vi "GE 5565PIORC.PIO.Scalar.vi"(11 "data type":T1) -> (0 "error out":errorcluster, 3 "pass?":bool)   [LabVIEW 2020]
uses:
  Typedefs/GE 5565PIORC.Data Types.ctl
  Source/GE 5565PIORC.lvclass/GE 5565PIORC.ctl
  Source/Methods/GE 5565PIORC.PIO.Write (Bool).vi
  Source/Methods/GE 5565PIORC.PIO.Read (Bool).vi
  Source/Methods/GE 5565PIORC.PIO.Write (SGL).vi
  Source/Methods/GE 5565PIORC.PIO.Read (SGL).vi
  Source/Methods/GE 5565PIORC.PIO.Write (DBL).vi
  Source/Methods/GE 5565PIORC.PIO.Read (DBL).vi
  Source/Methods/GE 5565PIORC.PIO.Write (I8).vi
  Source/Methods/GE 5565PIORC.PIO.Read (I8).vi
  Source/Methods/GE 5565PIORC.PIO.Write (I16).vi
  Source/Methods/GE 5565PIORC.PIO.Read (I16).vi
  Source/Methods/GE 5565PIORC.PIO.Write (I32).vi
  Source/Methods/GE 5565PIORC.PIO.Read (I32).vi
  Source/Methods/GE 5565PIORC.PIO.Write (I64).vi
  Source/Methods/GE 5565PIORC.PIO.Read (I64).vi
  Source/Methods/GE 5565PIORC.PIO.Write (U8).vi
  Source/Methods/GE 5565PIORC.PIO.Read (U8).vi
  Source/Methods/GE 5565PIORC.PIO.Write (U16).vi
  Source/Methods/GE 5565PIORC.PIO.Read (U16).vi
  Source/Methods/GE 5565PIORC.PIO.Write (U32).vi
  Source/Methods/GE 5565PIORC.PIO.Read (U32).vi
  Source/Methods/GE 5565PIORC.PIO.Write (U64).vi
  Source/Methods/GE 5565PIORC.PIO.Read (U64).vi
  Source/Methods/GE 5565PIORC.VISA.Move Out.vi
  Source/Methods/GE 5565PIORC.VISA.Move Out.String (U8).vi
  Source/Methods/GE 5565PIORC.VISA.Move In.vi
  Source/Methods/GE 5565PIORC.VISA.Move In.String (U8).vi
  Source/Methods/GE 5565PIORC.VISA.Return Handler.vi
  <vilib>/Utility/error.llb/Error Cluster From Error Code.vi
  Source/GE 5565PIORC.lvclass
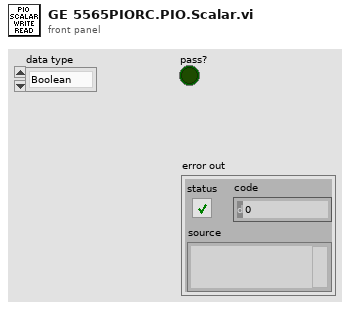
[diagram p1: front panel]
types:
  T1 = typedef "GE 5565PIORC.Data Types.ctl" = enum16{"Boolean", "Single", "Double", "I8", "I16", "I32", "I64", "U8", "U16", "U32", "U64"}
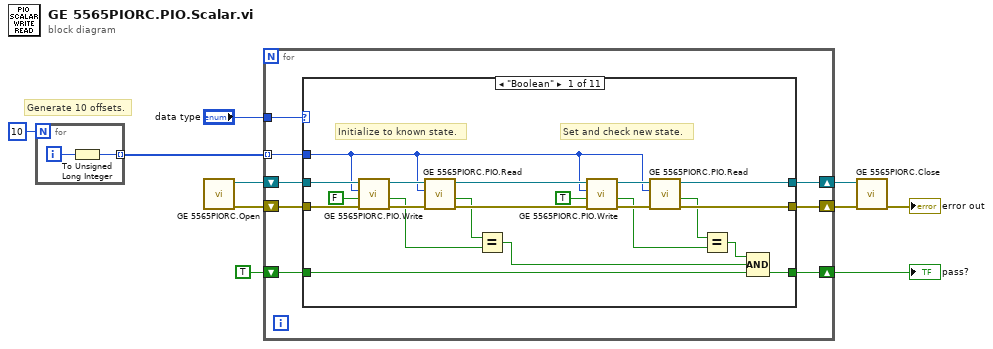
[diagram p0: block diagram]
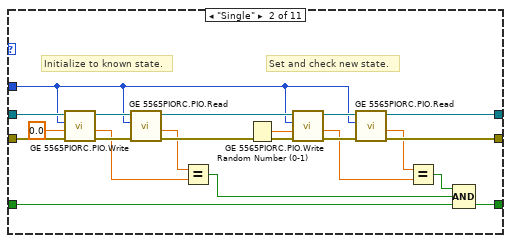
[diagram p2: hidden frame]
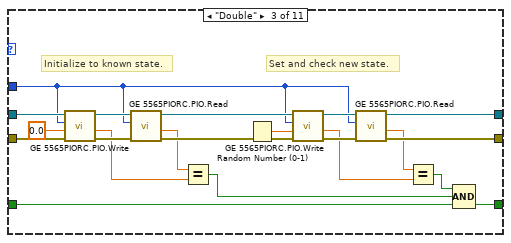
[diagram p3: hidden frame]
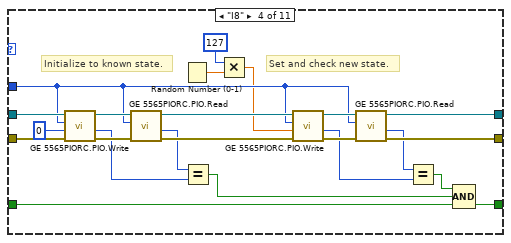
[diagram p4: hidden frame]
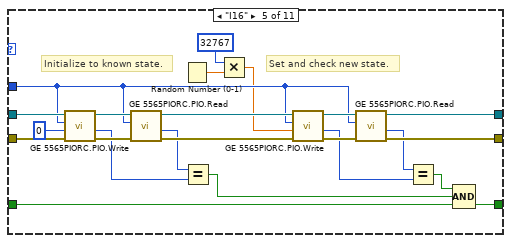
[diagram p5: hidden frame]
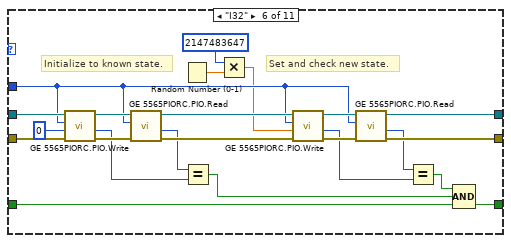
[diagram p6: hidden frame]
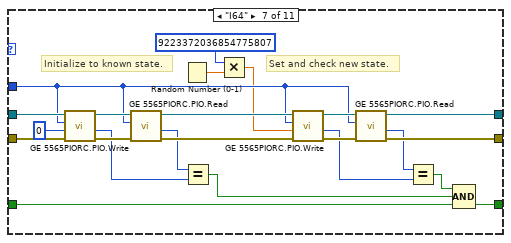
[diagram p7: hidden frame]
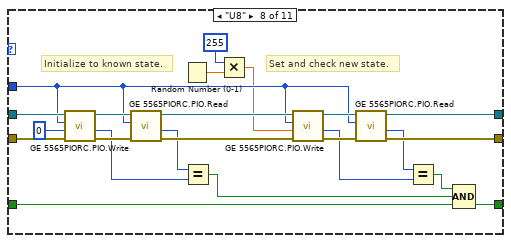
[diagram p8: hidden frame]
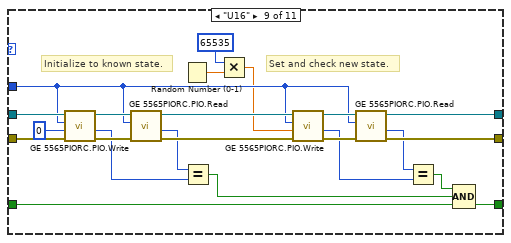
[diagram p9: hidden frame]
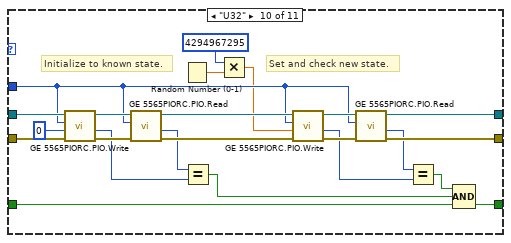
[diagram p10: hidden frame]
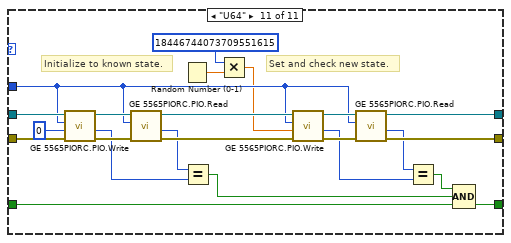
[diagram p11: hidden frame]
diagram:
  # "Generate 10 offsets."
  n1 = for {
    N: 10 -> [_]
    tunnel: [w12] -> w9 mode=indexing
    i -> [w11]
    n2 = To Unsigned Long Integer(number=w11) -> (unsigned 32bit integer=w12:u32)
  }
  n3 = call "GE 5565PIORC.Open.vi"() -> ("error out"=w5:errorcluster, "GE 5565PIORC"=w4:refnum<class "GE 5565PIORC.lvclass">)  [unwired: 10 in]
  n4 = for {
    tunnel: w9 -> [w19] mode=indexing
    tunnel: "data type" -> [w18]
    shift-right: [w14] -> w3
    shift-left: w4 -> [w20]
    shift-right: [w13] -> w2
    shift-left: w5 -> [w17]
    shift-right: [w15] -> w6
    shift-left: TRUE -> [w16]
    n5 = case shown="\"Boolean\"" w18 {
      tunnel: w20 -> [w41 w62 w83 w106 w129 w152 w175 w198 w221 w244 w267]
      tunnel: w19 -> [w21 w43 w64 w87 w110 w133 w156 w179 w202 w225 w248]
      tunnel: w17 -> [w40 w61 w82 w105 w128 w151 w174 w197 w220 w243 w266]
      tunnel: w16 -> [w34 w57 w78 w101 w124 w147 w170 w193 w216 w239 w262]
      tunnel: [w33 w56 w77 w100 w123 w146 w169 w192 w215 w238 w261] -> w15
      tunnel: [w32 w55 w76 w99 w122 w145 w168 w191 w214 w237 w260] -> w14
      tunnel: [w31 w54 w75 w98 w121 w144 w167 w190 w213 w236 w259] -> w13
      frame "Boolean" {
        # "Set and check new state."
        # "Initialize to known state."
        n6 = call-poly "GE 5565PIORC.PIO.Write.vi"("error in (no error)"=w40, "data"=FALSE, "offset"=w21, "GE 5565PIORC in"=w41) -> ("error out"=w37:errorcluster, "data out"=w30:bool, "GE 5565PIORC out"=w38:refnum<class "GE 5565PIORC.lvclass">)  [unwired: 5 in]
        n7 = call-poly "GE 5565PIORC.PIO.Read.vi"("error in (no error)"=w37, "offset"=w21, "GE 5565PIORC in"=w38) -> ("error out"=w36:errorcluster, "data"=w29:bool, "GE 5565PIORC out"=w35:refnum<class "GE 5565PIORC.lvclass">)  [unwired: 6 in]
        n8 = Equal?(x=w29, y=w30) -> (x = y?=w23:bool)
        n9 = call-poly "GE 5565PIORC.PIO.Write.vi"("error in (no error)"=w36, "data"=TRUE, "offset"=w21, "GE 5565PIORC in"=w35) -> ("error out"=w26:errorcluster, "data out"=w25:bool, "GE 5565PIORC out"=w27:refnum<class "GE 5565PIORC.lvclass">)  [unwired: 5 in]
        n10 = call-poly "GE 5565PIORC.PIO.Read.vi"("error in (no error)"=w26, "offset"=w21, "GE 5565PIORC in"=w27) -> ("error out"=w31:errorcluster, "data"=w24:bool, "GE 5565PIORC out"=w32:refnum<class "GE 5565PIORC.lvclass">)  [unwired: 6 in]
        n11 = Equal?(x=w24, y=w25) -> (x = y?=w22:bool)
        n12 = Compound Arithmetic op=AND(w22, w23, w34) -> (w33:bool)
      }
      frame "Single" {
        # "Set and check new state."
        # "Initialize to known state."
        n13 = call-poly "GE 5565PIORC.PIO.Write.vi"("error in (no error)"=w61, "data"=sgl 0.0, "offset"=w43, "GE 5565PIORC in"=w62) -> ("error out"=w59:errorcluster, "data out"=w53:sgl, "GE 5565PIORC out"=w60:refnum<class "GE 5565PIORC.lvclass">)  [unwired: 5 in]
        n14 = call-poly "GE 5565PIORC.PIO.Read.vi"("error in (no error)"=w59, "offset"=w43, "GE 5565PIORC in"=w60) -> ("error out"=w58:errorcluster, "data"=w52:sgl, "GE 5565PIORC out"=w44:refnum<class "GE 5565PIORC.lvclass">)  [unwired: 6 in]
        n15 = Equal?(x=w52, y=w53) -> (x = y?=w47:bool)
        n16 = Random Number (0-1)() -> (number: 0 to 1=w42:dbl)
        n17 = call-poly "GE 5565PIORC.PIO.Write.vi"("error in (no error)"=w58, "data"=w42, "offset"=w43, "GE 5565PIORC in"=w44) -> ("error out"=w50:errorcluster, "data out"=w49:sgl, "GE 5565PIORC out"=w51:refnum<class "GE 5565PIORC.lvclass">)  [unwired: 5 in]
        n18 = call-poly "GE 5565PIORC.PIO.Read.vi"("error in (no error)"=w50, "offset"=w43, "GE 5565PIORC in"=w51) -> ("error out"=w54:errorcluster, "data"=w48:sgl, "GE 5565PIORC out"=w55:refnum<class "GE 5565PIORC.lvclass">)  [unwired: 6 in]
        n19 = Equal?(x=w48, y=w49) -> (x = y?=w46:bool)
        n20 = Compound Arithmetic op=AND(w46, w47, w57) -> (w56:bool)
      }
      frame "Double" {
        # "Set and check new state."
        # "Initialize to known state."
        n21 = call-poly "GE 5565PIORC.PIO.Write.vi"("error in (no error)"=w82, "data"=0.0, "offset"=w64, "GE 5565PIORC in"=w83) -> ("error out"=w80:errorcluster, "data out"=w74:dbl, "GE 5565PIORC out"=w81:refnum<class "GE 5565PIORC.lvclass">)  [unwired: 5 in]
        n22 = call-poly "GE 5565PIORC.PIO.Read.vi"("error in (no error)"=w80, "offset"=w64, "GE 5565PIORC in"=w81) -> ("error out"=w79:errorcluster, "data"=w73:dbl, "GE 5565PIORC out"=w65:refnum<class "GE 5565PIORC.lvclass">)  [unwired: 6 in]
        n23 = Equal?(x=w73, y=w74) -> (x = y?=w68:bool)
        n24 = Random Number (0-1)() -> (number: 0 to 1=w63:dbl)
        n25 = call-poly "GE 5565PIORC.PIO.Write.vi"("error in (no error)"=w79, "data"=w63, "offset"=w64, "GE 5565PIORC in"=w65) -> ("error out"=w71:errorcluster, "data out"=w70:dbl, "GE 5565PIORC out"=w72:refnum<class "GE 5565PIORC.lvclass">)  [unwired: 5 in]
        n26 = call-poly "GE 5565PIORC.PIO.Read.vi"("error in (no error)"=w71, "offset"=w64, "GE 5565PIORC in"=w72) -> ("error out"=w75:errorcluster, "data"=w69:dbl, "GE 5565PIORC out"=w76:refnum<class "GE 5565PIORC.lvclass">)  [unwired: 6 in]
        n27 = Equal?(x=w69, y=w70) -> (x = y?=w67:bool)
        n28 = Compound Arithmetic op=AND(w67, w68, w78) -> (w77:bool)
      }
      frame "I8" {
        # "Set and check new state."
        # "Initialize to known state."
        n29 = call-poly "GE 5565PIORC.PIO.Write.vi"("error in (no error)"=w105, "data"=i8 0, "offset"=w87, "GE 5565PIORC in"=w106) -> ("error out"=w103:errorcluster, "data out"=w97:i8, "GE 5565PIORC out"=w104:refnum<class "GE 5565PIORC.lvclass">)  [unwired: 5 in]
        n30 = call-poly "GE 5565PIORC.PIO.Read.vi"("error in (no error)"=w103, "offset"=w87, "GE 5565PIORC in"=w104) -> ("error out"=w102:errorcluster, "data"=w96:i8, "GE 5565PIORC out"=w88:refnum<class "GE 5565PIORC.lvclass">)  [unwired: 6 in]
        n31 = Random Number (0-1)() -> (number: 0 to 1=w86:dbl)
        n32 = Equal?(x=w96, y=w97) -> (x = y?=w91:bool)
        n33 = Multiply(x=i8 127, y=w86) -> (x*y=w84:dbl)
        n34 = call-poly "GE 5565PIORC.PIO.Write.vi"("error in (no error)"=w102, "data"=w84, "offset"=w87, "GE 5565PIORC in"=w88) -> ("error out"=w94:errorcluster, "data out"=w93:i8, "GE 5565PIORC out"=w95:refnum<class "GE 5565PIORC.lvclass">)  [unwired: 5 in]
        n35 = call-poly "GE 5565PIORC.PIO.Read.vi"("error in (no error)"=w94, "offset"=w87, "GE 5565PIORC in"=w95) -> ("error out"=w98:errorcluster, "data"=w92:i8, "GE 5565PIORC out"=w99:refnum<class "GE 5565PIORC.lvclass">)  [unwired: 6 in]
        n36 = Equal?(x=w92, y=w93) -> (x = y?=w90:bool)
        n37 = Compound Arithmetic op=AND(w90, w91, w101) -> (w100:bool)
      }
      frame "I16" {
        # "Set and check new state."
        # "Initialize to known state."
        n38 = call-poly "GE 5565PIORC.PIO.Write.vi"("error in (no error)"=w128, "data"=i16 0, "offset"=w110, "GE 5565PIORC in"=w129) -> ("error out"=w126:errorcluster, "data out"=w120:i16, "GE 5565PIORC out"=w127:refnum<class "GE 5565PIORC.lvclass">)  [unwired: 5 in]
        n39 = call-poly "GE 5565PIORC.PIO.Read.vi"("error in (no error)"=w126, "offset"=w110, "GE 5565PIORC in"=w127) -> ("error out"=w125:errorcluster, "data"=w119:i16, "GE 5565PIORC out"=w111:refnum<class "GE 5565PIORC.lvclass">)  [unwired: 6 in]
        n40 = Random Number (0-1)() -> (number: 0 to 1=w109:dbl)
        n41 = Equal?(x=w119, y=w120) -> (x = y?=w114:bool)
        n42 = Multiply(x=i16 32767, y=w109) -> (x*y=w107:dbl)
        n43 = call-poly "GE 5565PIORC.PIO.Write.vi"("error in (no error)"=w125, "data"=w107, "offset"=w110, "GE 5565PIORC in"=w111) -> ("error out"=w117:errorcluster, "data out"=w116:i16, "GE 5565PIORC out"=w118:refnum<class "GE 5565PIORC.lvclass">)  [unwired: 5 in]
        n44 = call-poly "GE 5565PIORC.PIO.Read.vi"("error in (no error)"=w117, "offset"=w110, "GE 5565PIORC in"=w118) -> ("error out"=w121:errorcluster, "data"=w115:i16, "GE 5565PIORC out"=w122:refnum<class "GE 5565PIORC.lvclass">)  [unwired: 6 in]
        n45 = Equal?(x=w115, y=w116) -> (x = y?=w113:bool)
        n46 = Compound Arithmetic op=AND(w113, w114, w124) -> (w123:bool)
      }
      frame "I32" {
        # "Set and check new state."
        # "Initialize to known state."
        n47 = call-poly "GE 5565PIORC.PIO.Write.vi"("error in (no error)"=w151, "data"=0, "offset"=w133, "GE 5565PIORC in"=w152) -> ("error out"=w149:errorcluster, "data out"=w143:i32, "GE 5565PIORC out"=w150:refnum<class "GE 5565PIORC.lvclass">)  [unwired: 5 in]
        n48 = call-poly "GE 5565PIORC.PIO.Read.vi"("error in (no error)"=w149, "offset"=w133, "GE 5565PIORC in"=w150) -> ("error out"=w148:errorcluster, "data"=w142:i32, "GE 5565PIORC out"=w134:refnum<class "GE 5565PIORC.lvclass">)  [unwired: 6 in]
        n49 = Random Number (0-1)() -> (number: 0 to 1=w132:dbl)
        n50 = Equal?(x=w142, y=w143) -> (x = y?=w137:bool)
        n51 = Multiply(x=2147483647, y=w132) -> (x*y=w130:dbl)
        n52 = call-poly "GE 5565PIORC.PIO.Write.vi"("error in (no error)"=w148, "data"=w130, "offset"=w133, "GE 5565PIORC in"=w134) -> ("error out"=w140:errorcluster, "data out"=w139:i32, "GE 5565PIORC out"=w141:refnum<class "GE 5565PIORC.lvclass">)  [unwired: 5 in]
        n53 = call-poly "GE 5565PIORC.PIO.Read.vi"("error in (no error)"=w140, "offset"=w133, "GE 5565PIORC in"=w141) -> ("error out"=w144:errorcluster, "data"=w138:i32, "GE 5565PIORC out"=w145:refnum<class "GE 5565PIORC.lvclass">)  [unwired: 6 in]
        n54 = Equal?(x=w138, y=w139) -> (x = y?=w136:bool)
        n55 = Compound Arithmetic op=AND(w136, w137, w147) -> (w146:bool)
      }
      frame "I64" {
        # "Set and check new state."
        # "Initialize to known state."
        n56 = call-poly "GE 5565PIORC.PIO.Write.vi"("error in (no error)"=w174, "data"=i64 0, "offset"=w156, "GE 5565PIORC in"=w175) -> ("error out"=w172:errorcluster, "data out"=w166:i64, "GE 5565PIORC out"=w173:refnum<class "GE 5565PIORC.lvclass">)  [unwired: 5 in]
        n57 = call-poly "GE 5565PIORC.PIO.Read.vi"("error in (no error)"=w172, "offset"=w156, "GE 5565PIORC in"=w173) -> ("error out"=w171:errorcluster, "data"=w165:i64, "GE 5565PIORC out"=w157:refnum<class "GE 5565PIORC.lvclass">)  [unwired: 6 in]
        n58 = Random Number (0-1)() -> (number: 0 to 1=w155:dbl)
        n59 = Equal?(x=w165, y=w166) -> (x = y?=w160:bool)
        n60 = Multiply(x=i64 9223372036854775807, y=w155) -> (x*y=w153:dbl)
        n61 = call-poly "GE 5565PIORC.PIO.Write.vi"("error in (no error)"=w171, "data"=w153, "offset"=w156, "GE 5565PIORC in"=w157) -> ("error out"=w163:errorcluster, "data out"=w162:i64, "GE 5565PIORC out"=w164:refnum<class "GE 5565PIORC.lvclass">)  [unwired: 5 in]
        n62 = call-poly "GE 5565PIORC.PIO.Read.vi"("error in (no error)"=w163, "offset"=w156, "GE 5565PIORC in"=w164) -> ("error out"=w167:errorcluster, "data"=w161:i64, "GE 5565PIORC out"=w168:refnum<class "GE 5565PIORC.lvclass">)  [unwired: 6 in]
        n63 = Equal?(x=w161, y=w162) -> (x = y?=w159:bool)
        n64 = Compound Arithmetic op=AND(w159, w160, w170) -> (w169:bool)
      }
      frame "U8" {
        # "Set and check new state."
        # "Initialize to known state."
        n65 = call-poly "GE 5565PIORC.PIO.Write.vi"("error in (no error)"=w197, "data"=u8 0, "offset"=w179, "GE 5565PIORC in"=w198) -> ("error out"=w195:errorcluster, "data out"=w189:u8, "GE 5565PIORC out"=w196:refnum<class "GE 5565PIORC.lvclass">)  [unwired: 5 in]
        n66 = call-poly "GE 5565PIORC.PIO.Read.vi"("error in (no error)"=w195, "offset"=w179, "GE 5565PIORC in"=w196) -> ("error out"=w194:errorcluster, "data"=w188:u8, "GE 5565PIORC out"=w180:refnum<class "GE 5565PIORC.lvclass">)  [unwired: 6 in]
        n67 = Random Number (0-1)() -> (number: 0 to 1=w178:dbl)
        n68 = Equal?(x=w188, y=w189) -> (x = y?=w183:bool)
        n69 = Multiply(x=u8 255, y=w178) -> (x*y=w176:dbl)
        n70 = call-poly "GE 5565PIORC.PIO.Write.vi"("error in (no error)"=w194, "data"=w176, "offset"=w179, "GE 5565PIORC in"=w180) -> ("error out"=w186:errorcluster, "data out"=w185:u8, "GE 5565PIORC out"=w187:refnum<class "GE 5565PIORC.lvclass">)  [unwired: 5 in]
        n71 = call-poly "GE 5565PIORC.PIO.Read.vi"("error in (no error)"=w186, "offset"=w179, "GE 5565PIORC in"=w187) -> ("error out"=w190:errorcluster, "data"=w184:u8, "GE 5565PIORC out"=w191:refnum<class "GE 5565PIORC.lvclass">)  [unwired: 6 in]
        n72 = Equal?(x=w184, y=w185) -> (x = y?=w182:bool)
        n73 = Compound Arithmetic op=AND(w182, w183, w193) -> (w192:bool)
      }
      frame "U16" {
        # "Set and check new state."
        # "Initialize to known state."
        n74 = call-poly "GE 5565PIORC.PIO.Write.vi"("error in (no error)"=w220, "data"=u16 0, "offset"=w202, "GE 5565PIORC in"=w221) -> ("error out"=w218:errorcluster, "data out"=w212:u16, "GE 5565PIORC out"=w219:refnum<class "GE 5565PIORC.lvclass">)  [unwired: 5 in]
        n75 = call-poly "GE 5565PIORC.PIO.Read.vi"("error in (no error)"=w218, "offset"=w202, "GE 5565PIORC in"=w219) -> ("error out"=w217:errorcluster, "data"=w211:u16, "GE 5565PIORC out"=w203:refnum<class "GE 5565PIORC.lvclass">)  [unwired: 6 in]
        n76 = Random Number (0-1)() -> (number: 0 to 1=w201:dbl)
        n77 = Equal?(x=w211, y=w212) -> (x = y?=w206:bool)
        n78 = Multiply(x=u16 65535, y=w201) -> (x*y=w199:dbl)
        n79 = call-poly "GE 5565PIORC.PIO.Write.vi"("error in (no error)"=w217, "data"=w199, "offset"=w202, "GE 5565PIORC in"=w203) -> ("error out"=w209:errorcluster, "data out"=w208:u16, "GE 5565PIORC out"=w210:refnum<class "GE 5565PIORC.lvclass">)  [unwired: 5 in]
        n80 = call-poly "GE 5565PIORC.PIO.Read.vi"("error in (no error)"=w209, "offset"=w202, "GE 5565PIORC in"=w210) -> ("error out"=w213:errorcluster, "data"=w207:u16, "GE 5565PIORC out"=w214:refnum<class "GE 5565PIORC.lvclass">)  [unwired: 6 in]
        n81 = Equal?(x=w207, y=w208) -> (x = y?=w205:bool)
        n82 = Compound Arithmetic op=AND(w205, w206, w216) -> (w215:bool)
      }
      frame "U32" {
        # "Set and check new state."
        # "Initialize to known state."
        n83 = call-poly "GE 5565PIORC.PIO.Write.vi"("error in (no error)"=w243, "data"=u32 0, "offset"=w225, "GE 5565PIORC in"=w244) -> ("error out"=w241:errorcluster, "data out"=w235:u32, "GE 5565PIORC out"=w242:refnum<class "GE 5565PIORC.lvclass">)  [unwired: 5 in]
        n84 = call-poly "GE 5565PIORC.PIO.Read.vi"("error in (no error)"=w241, "offset"=w225, "GE 5565PIORC in"=w242) -> ("error out"=w240:errorcluster, "data"=w234:u32, "GE 5565PIORC out"=w226:refnum<class "GE 5565PIORC.lvclass">)  [unwired: 6 in]
        n85 = Random Number (0-1)() -> (number: 0 to 1=w224:dbl)
        n86 = Equal?(x=w234, y=w235) -> (x = y?=w229:bool)
        n87 = Multiply(x=u32 4294967295, y=w224) -> (x*y=w222:dbl)
        n88 = call-poly "GE 5565PIORC.PIO.Write.vi"("error in (no error)"=w240, "data"=w222, "offset"=w225, "GE 5565PIORC in"=w226) -> ("error out"=w232:errorcluster, "data out"=w231:u32, "GE 5565PIORC out"=w233:refnum<class "GE 5565PIORC.lvclass">)  [unwired: 5 in]
        n89 = call-poly "GE 5565PIORC.PIO.Read.vi"("error in (no error)"=w232, "offset"=w225, "GE 5565PIORC in"=w233) -> ("error out"=w236:errorcluster, "data"=w230:u32, "GE 5565PIORC out"=w237:refnum<class "GE 5565PIORC.lvclass">)  [unwired: 6 in]
        n90 = Equal?(x=w230, y=w231) -> (x = y?=w228:bool)
        n91 = Compound Arithmetic op=AND(w228, w229, w239) -> (w238:bool)
      }
      frame "U64" {
        # "Set and check new state."
        # "Initialize to known state."
        n92 = call-poly "GE 5565PIORC.PIO.Write.vi"("error in (no error)"=w266, "data"=u64 0, "offset"=w248, "GE 5565PIORC in"=w267) -> ("error out"=w264:errorcluster, "data out"=w258:u64, "GE 5565PIORC out"=w265:refnum<class "GE 5565PIORC.lvclass">)  [unwired: 5 in]
        n93 = call-poly "GE 5565PIORC.PIO.Read.vi"("error in (no error)"=w264, "offset"=w248, "GE 5565PIORC in"=w265) -> ("error out"=w263:errorcluster, "data"=w257:u64, "GE 5565PIORC out"=w249:refnum<class "GE 5565PIORC.lvclass">)  [unwired: 6 in]
        n94 = Random Number (0-1)() -> (number: 0 to 1=w247:dbl)
        n95 = Equal?(x=w257, y=w258) -> (x = y?=w252:bool)
        n96 = Multiply(x=u64 18446744073709551615, y=w247) -> (x*y=w245:dbl)
        n97 = call-poly "GE 5565PIORC.PIO.Write.vi"("error in (no error)"=w263, "data"=w245, "offset"=w248, "GE 5565PIORC in"=w249) -> ("error out"=w255:errorcluster, "data out"=w254:u64, "GE 5565PIORC out"=w256:refnum<class "GE 5565PIORC.lvclass">)  [unwired: 5 in]
        n98 = call-poly "GE 5565PIORC.PIO.Read.vi"("error in (no error)"=w255, "offset"=w248, "GE 5565PIORC in"=w256) -> ("error out"=w259:errorcluster, "data"=w253:u64, "GE 5565PIORC out"=w260:refnum<class "GE 5565PIORC.lvclass">)  [unwired: 6 in]
        n99 = Equal?(x=w253, y=w254) -> (x = y?=w251:bool)
        n100 = Compound Arithmetic op=AND(w251, w252, w262) -> (w261:bool)
      }
    }
  }
  "pass?" <- w6
  n101 = call "GE 5565PIORC.Close.vi"("error in (no error)"=w2, "GE 5565PIORC"=w3) -> ("error out"=→"error out":errorcluster)  [unwired: 9 in]
